vi "imageProfile.vi"(8 "error in (no error)":errorcluster, 10 "Point":T1, 11 "ImageStreamViewer in":refnum<class "ImageStreamViewer.lvclass">) -> (0 "error out":errorcluster, 3 "ImageStreamViewer out":refnum<class "ImageStreamViewer.lvclass">)   [LabVIEW 2009, in "Views.lvlib" / "Camera.lvlib" / "ImageStreamViewer.lvclass"]
uses:
  ImageStreamViewer.lvclass
  <vilib>/Utility/miscctls.llb/LVPoint32TypeDef.ctl
  ImageStreamViewer.lvclass/ImageStreamViewer.ctl
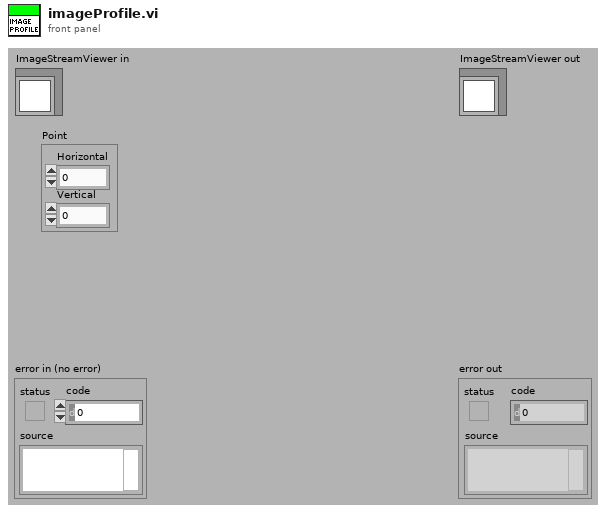
[diagram p1: front panel]
types:
  T1 = typedef "LVPoint32TypeDef.ctl" = cluster{"Horizontal":i32, "Vertical":i32}
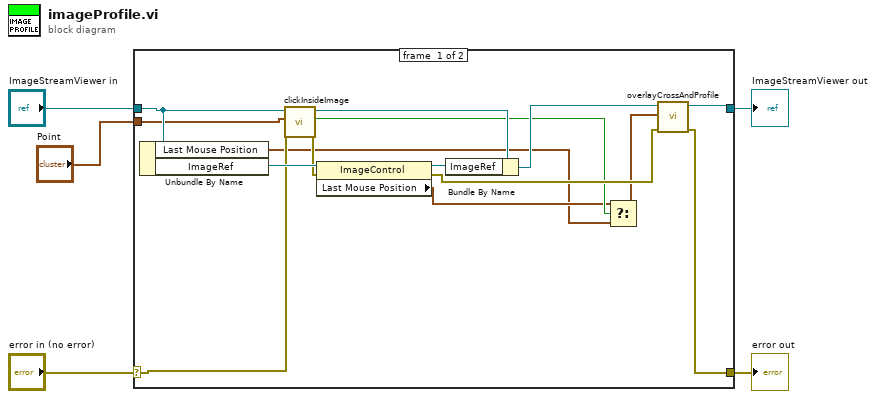
[diagram p0: block diagram]
diagram:
  n1 = case shown="No Error" "error in (no error)" {
    selector: "error in (no error)" -> [w11 w22]
    tunnel: [w16 w22] -> w4
    tunnel: [w15 w21] -> w2
    tunnel: "ImageStreamViewer in" -> [w13 w21]
    tunnel: "Point" -> [w6 _]
    frame #0 {
      n2 = Unbundle By Name(w13) -> ("Last Mouse Position"=w7:cluster{"X":i32, "Y":i32}, "ImageRef"=w20:refnum<vi>)
      n3 = call "clickInsideImage.vi"("error in (no error)"=w11, "Point"=w6, "ImageStreamViewer in"=w13) -> ("error out"=w9:errorcluster, "clickInsideImage?"=w10:bool, "ImageStreamViewer out"=w12:refnum<class "ImageStreamViewer.lvclass">)  [unwired: 6 in]
      n4 = property class="ImageControl"(reference=w20, error in=w9) -> (reference out=w19:refnum<vi>, error out=w17:errorcluster, "Last Mouse Position"=w8:cluster{"X":i32, "Y":i32})
      n5 = Bundle By Name(cluster=w12, "ImageRef"=w19) -> (w18:refnum<class "ImageStreamViewer.lvclass">)
      n6 = Select(t=w8, s=w10, f=w7) -> (s? t:f=w14:cluster{"X":i32, "Y":i32})
      n7 = call "overlayCrossAndProfile.vi"("error in (no error)"=w17, "Last Mouse P"=w14, "ImageStreamViewer in"=w18) -> ("error out"=w16:errorcluster, "ImageStreamViewer out"=w15:refnum<class "ImageStreamViewer.lvclass">)  [unwired: 7 in]
    }
    frame #1 {
    }
  }
  "error out" <- w4
  "ImageStreamViewer out" <- w2
